vi "Copy from start.vi"(1 "length":i32=-1, 2 "bytestream":refnum<class "Bytestream.lvclass">) -> (0 "data":u8[](array[numeric]) format="%02x")   [LabVIEW 2020, in "NI_Bytestream.lvlib" / "Bytestream.lvclass"]
uses:
  <vilib>/Array/Bytestream/Bytestream.lvclass
  <vilib>/Array/Bytestream/Bytestream.lvclass/Bytestream.ctl
  <vilib>/Array/Bytestream/Get Logical Datum.vi
  <vilib>/Array/Bytestream/Datum Size.vi
  <vilib>/Array/Bytestream/Count Datums.vi
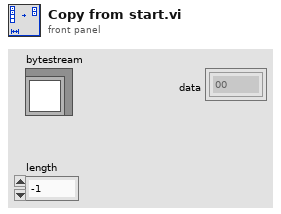
[diagram p1: front panel]
types:
  T1 = typedef "NI_Bytestream.lvlib/Bytestream.lvclass/Datum.ctl" = cluster{"array":u8[], "index":i32}
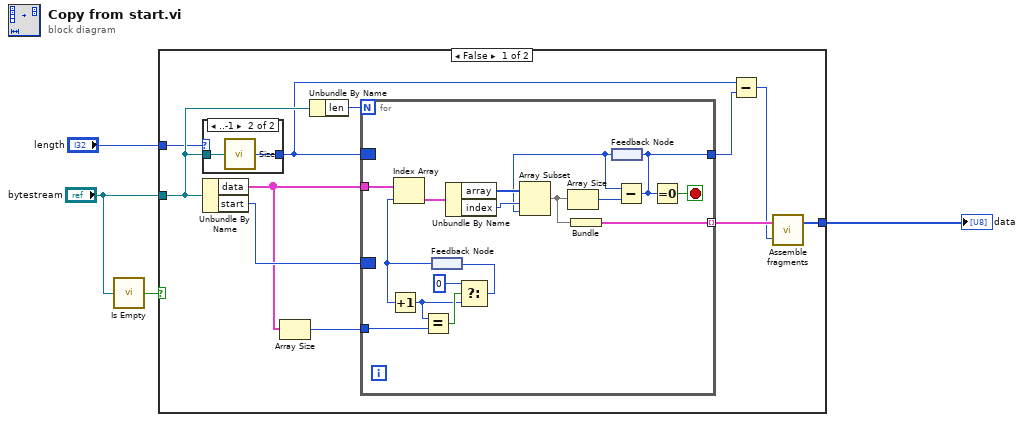
[diagram p0: block diagram]
diagram:
  n1 = call <vilib>:"Is Empty.vi"("a"="bytestream") -> ("empty?"=w1:bool)
  n2 = case shown="False" w1 {
    tunnel: "length" -> [w6 _]
    tunnel: [w13 _] -> w3
    tunnel: "bytestream" -> [w7 _]
    frame False {
      n3 = case shown="..-1" w6 {
        selector: w6 -> [w32 _]
        tunnel: w7 -> [_ w34]
        tunnel: [w32 w33] -> w5
        frame Default {
        }
        frame ..-1 {
          n4 = call <vilib>:"Size.vi"("ByteArrayTuple in"=w34) -> ("size"=w33:i32)
        }
      }
      n5 = Unbundle By Name(w7) -> ("data"=w11:T1[], "start"=w12:i32)
      n6 = Array Size(array=w11) -> (size(s)=w10:i32)
      n7 = Unbundle By Name(w7) -> ("len"=w9:i32)
      n8 = for {
        N: w9 -> [_]
        tunnel: [w30] -> w15 mode=indexing
        tunnel: w11 -> [w28]
        tunnel: w10 -> [w27]
        border: w5 -> [_]
        tunnel: [w16] -> w8
        border: w12 -> [_]
        stop <- w31 stop-if-true
        n9 = feedback #1() -> (w22:i32)
        n10 = Increment(x=w22) -> (x+1=w25:i32)
        n11 = Index Array(array=w28, index=w22) -> (element=w19:T1)
        n12 = Equal?(x=w25, y=w27) -> (x = y?=w26:bool)
        n13 = Unbundle By Name(w19) -> ("array"=w21:u8[], "index"=w20:i32)
        n14 = Select(t=0, s=w26, f=w25) -> (s? t:f=w23:i32)
        n15 = feedback-in #1(w23) -> ()
        n16 = feedback #2() -> (w18:i32)
        n17 = Array Subset(array=w21, index=w20, length=w18) -> (w17:u8[])
        n18 = Array Size(array=w17) -> (size(s)=w29:i32)
        n19 = Bundle(w17) -> (w30:cluster{u8[]})  [unwired: 1 in]
        n20 = Subtract(x=w18, y=w29) -> (x-y=w16:i32)
        n21 = feedback-in #2(w16) -> ()
        n22 = Equal To 0?(x=w16) -> (x = 0?=w31:bool)
      }
      n23 = Subtract(x=w5, y=w8) -> (x-y=w14:i32)
      n24 = call <vilib>:"Assemble fragments.vi"("Numeric"=w14, "Array in"=w15) -> ("Array out"=w13:u8[])  [unwired: 1 in]
    }
    frame True {
    }
  }
  "data" <- w3
